vi "DAQInit.vi"(6 "Scan/Meas Parameters":T5={"Pixel Dwell Time (s)"=0.0001, "Pixel Size"=200.0, "X Min (V)"=-7.5, "X Max (V)"=7.5, "Y Min (V)"=-7.5, "Y Max (V)"=7.5, "XY Factor (1/V)"=0.2}, 7 "Calibration Parameters":T4={"Target Lifetime (s)"=4e-09, "Integration Time (s)"=0.1, "Calibration Steps"=500.0}, 8 "error in":errorcluster, 9 "Functions":T6(ring)=enum."Measurement", 10 "Global Parameters":T1={"DC AI Min (V)"=0.0015, "DC AI Max (V)"=0.06, "Mixer AI Min (V)"=-0.3, "Mixer AI Max (V)"=0.3, "Bias AO Min (V)"=-1.0, "Bias AO Max (V)"=7.0, "Scan AO Min (V)"=-10.0, "Scan AO Max (V)"=10.0, "Fast Samp Freq (Hz)"=2500000.0, "Slow Samp Freq (Hz)"=250000.0}, 11 "DAQ Channels":T3) -> (0 "error out":errorcluster, 2 "Expected Time (s)":dbl=98.154, 3 "Tasks Out":T2)   [LabVIEW 2015]
uses:
  <vilib>/DAQmx/create/channels.llb/DAQmx Create Channel (AO-Voltage-Basic).vi
  <vilib>/DAQmx/configure/timing.llb/DAQmx Timing (Sample Clock).vi
  <vilib>/DAQmx/create/channels.llb/DAQmx Create Channel (AI-Voltage-Basic).vi
  <vilib>/DAQmx/configure/trigger.llb/DAQmx Start Trigger (Digital Edge).vi
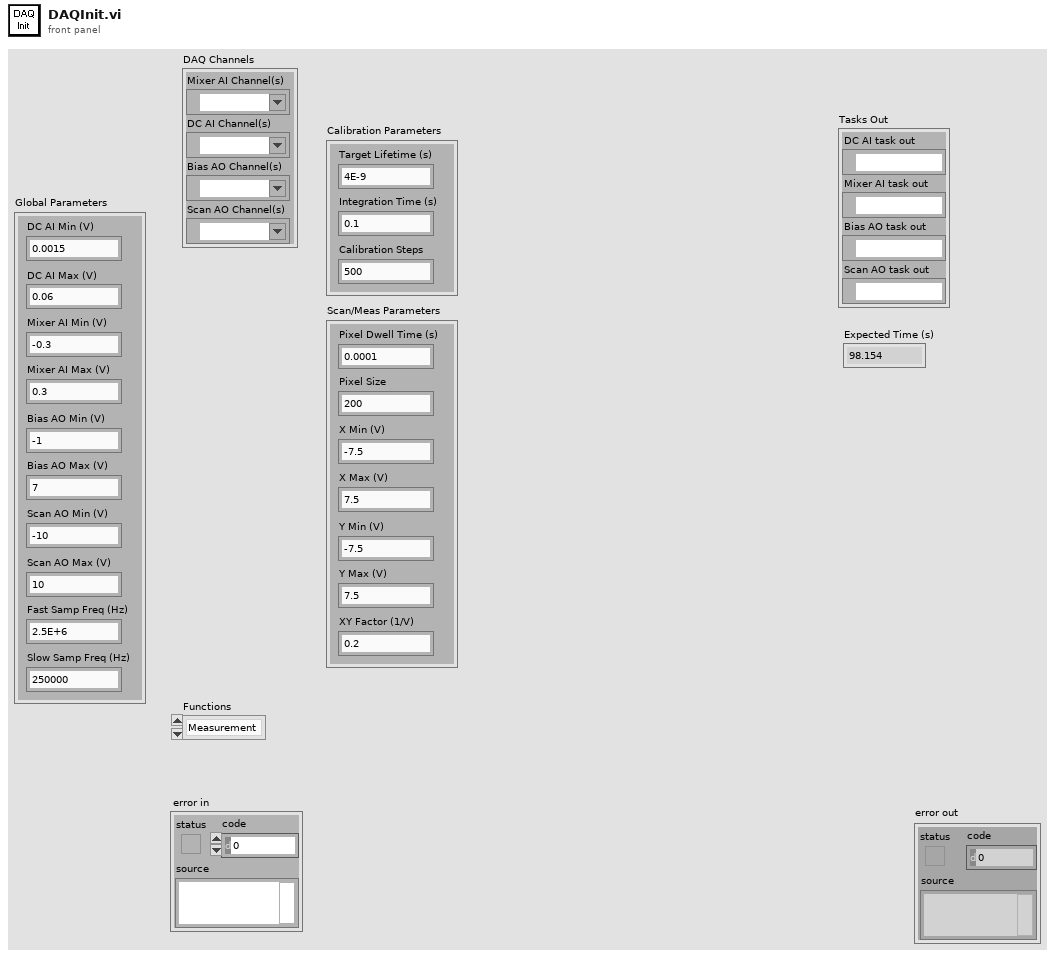
[diagram p1: front panel]
types:
  T1 = cluster{"DC AI Min (V)":dbl, "DC AI Max (V)":dbl, "Mixer AI Min (V)":dbl, "Mixer AI Max (V)":dbl, "Bias AO Min (V)":dbl, "Bias AO Max (V)":dbl, "Scan AO Min (V)":dbl, "Scan AO Max (V)":dbl, "Fast Samp Freq (Hz)":dbl, "Slow Samp Freq (Hz)":dbl}
  T2 = cluster{"DC AI task out":refnum<k21>, "Mixer AI task out":refnum<k21>, "Bias AO task out":refnum<k21>, "Scan AO task out":refnum<k21>}
  T3 = cluster{"Mixer AI Channel(s)":tag, "DC AI Channel(s)":tag, "Bias AO Channel(s) ":tag, "Scan AO Channel(s)":tag}
  T4 = cluster{"Target Lifetime (s)":dbl, "Integration Time (s)":dbl, "Calibration Steps":dbl}
  T5 = cluster{"Pixel Dwell Time (s)":dbl, "Pixel Size":dbl, "X Min (V)":dbl, "X Max (V)":dbl, "Y Min (V)":dbl, "Y Max (V)":dbl, "XY Factor (1/V)":dbl}
  T6 = enum32{"Calibration", "Fast Scan", "Measurement"}
  T7 = cluster{"task out":refnum<k21>, "task out":refnum<k21>, "task out":refnum<k21>, "task out":refnum<k21>}
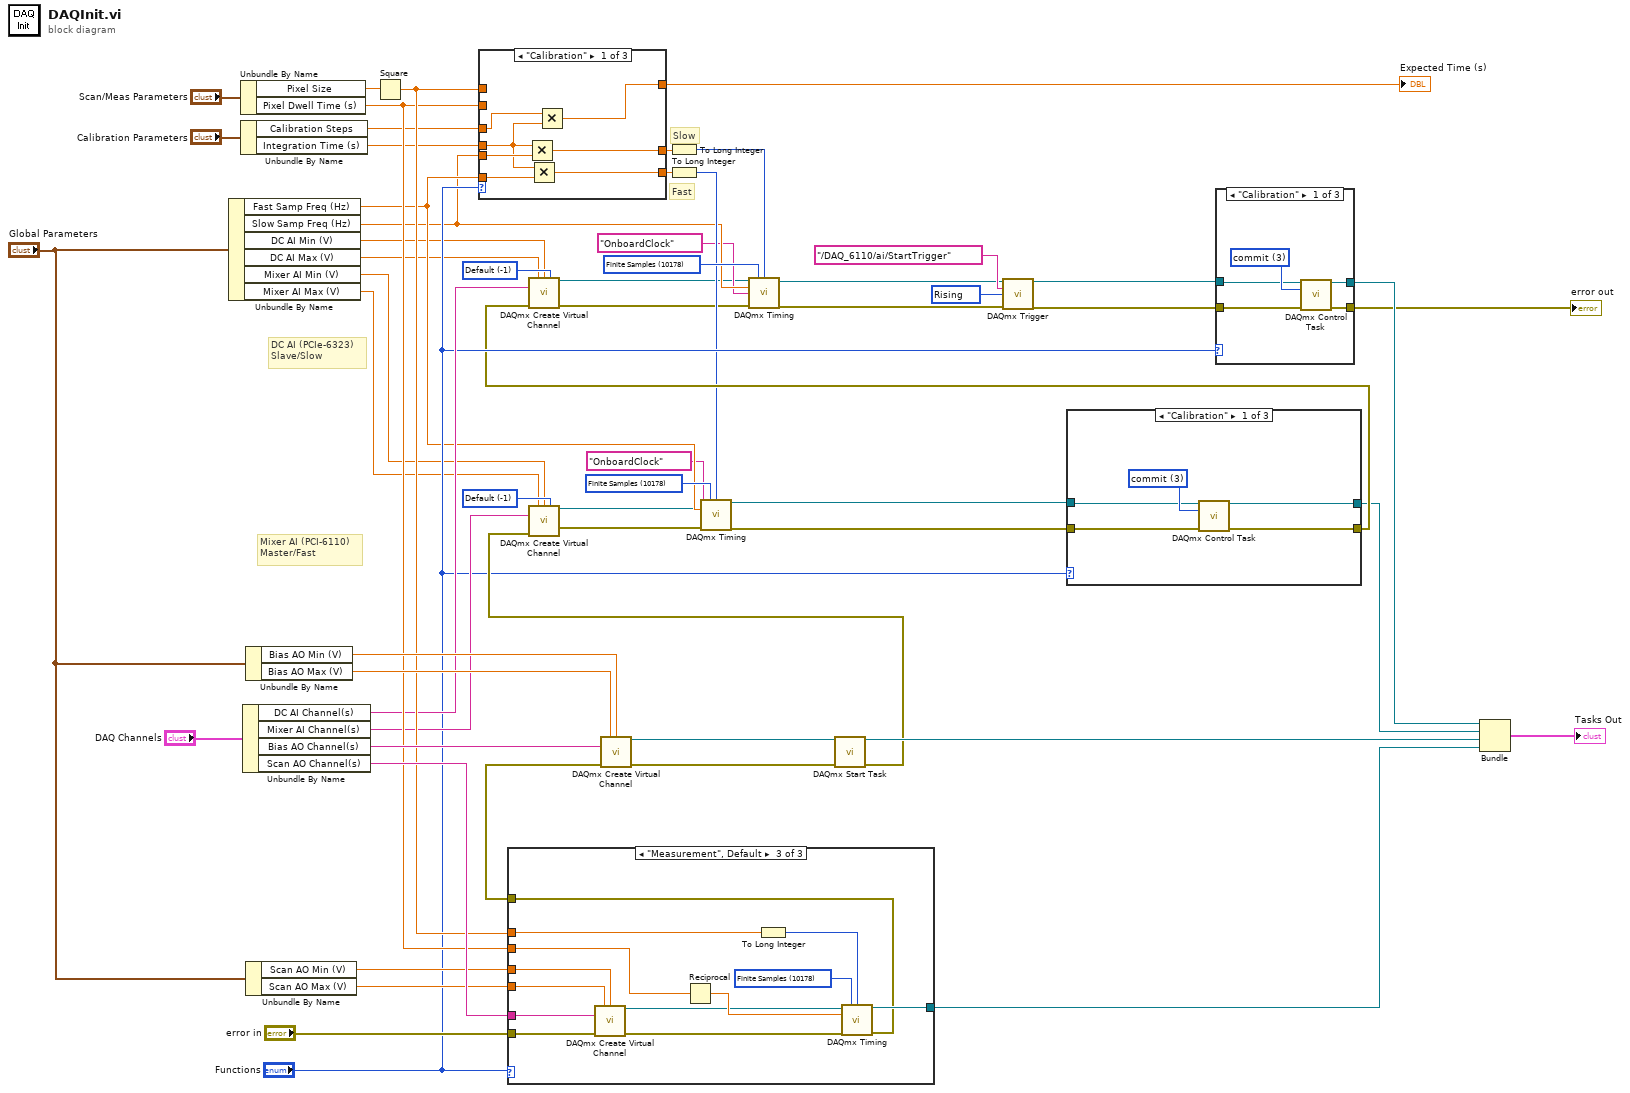
[diagram p0: block diagram]
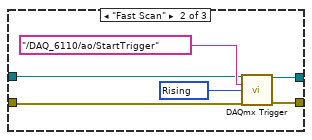
[diagram p2: hidden frame]
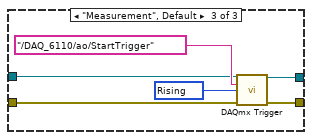
[diagram p3: hidden frame]
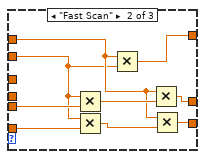
[diagram p4: hidden frame]
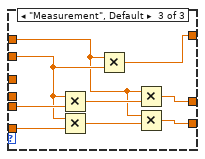
[diagram p5: hidden frame]
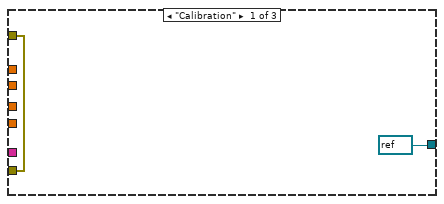
[diagram p8: hidden frame]
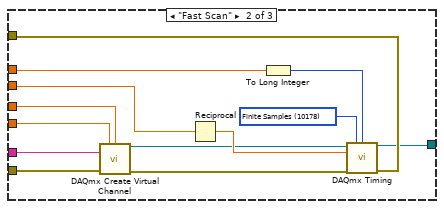
[diagram p9: hidden frame]
diagram:
  w13 = 10280 items=["Rising"=10280, "Falling"=10171] ("edge")
  w34 = 10178 items=["Finite Samples"=10178, "Continuous Samples"=10123, "Hardware Timed Single Point"=12522] ("sample mode")
  w35 = -1 items=["Default"=-1, "RSE"=10083, "NRSE"=10078, "Differential"=10106, "Pseudodifferential"=12529] ("input terminal configuration")
  w43 = 10178 items=["Finite Samples"=10178, "Continuous Samples"=10123, "Hardware Timed Single Point"=12522] ("sample mode")
  w44 = -1 items=["Default"=-1, "RSE"=10083, "NRSE"=10078, "Differential"=10106, "Pseudodifferential"=12529] ("input terminal configuration")
  # "Fast"
  # "Slow"
  # "DC AI (PCIe-6323)\nSlave/Slow"
  # "Mixer AI (PCI-6110)\nMaster/Fast"
  n1 = Unbundle By Name("Global Parameters") -> ("Fast Samp Freq (Hz)"=w24:dbl, "Slow Samp Freq (Hz)"=w20:dbl, "DC AI Min (V)"=w4:dbl, "DC AI Max (V)"=w2:dbl, "Mixer AI Min (V)"=w3:dbl, "Mixer AI Max (V)"=w1:dbl)
  n2 = Unbundle By Name("Scan/Meas Parameters") -> ("Pixel Size"=w53:dbl, "Pixel Dwell Time (s)"=w41:dbl)
  n3 = Unbundle By Name("Calibration Parameters") -> ("Calibration Steps"=w37:dbl, "Integration Time (s)"=w39:dbl)
  n4 = Unbundle By Name("DAQ Channels") -> ("DC AI Channel(s)"=w31:tag, "Mixer AI Channel(s)"=w32:tag, "Bias AO Channel(s)"=w48:tag, "Scan AO Channel(s)"=w56:tag)
  n5 = Unbundle By Name("Global Parameters") -> ("Bias AO Min (V)"=w46:dbl, "Bias AO Max (V)"=w47:dbl)
  n6 = Unbundle By Name("Global Parameters") -> ("Scan AO Min (V)"=w54:dbl, "Scan AO Max (V)"=w55:dbl)
  n7 = Square(x=w53) -> (x^2=w42:dbl)
  n8 = case shown="\"Calibration\"" "Functions" {
    tunnel: w20 -> [w66 w70 w83]
    tunnel: w42 -> [_ w71 w76]
    tunnel: w41 -> [_ w68 w79]
    tunnel: [w65 w74 w82] -> w40
    tunnel: w39 -> [w62 _ _]
    tunnel: [w63 w73 w81] -> w38
    tunnel: w37 -> [w64 _ _]
    tunnel: w24 -> [w61 w69 w80]
    tunnel: [w60 w72 w78] -> w26
    frame "Calibration" {
      n9 = Multiply(x=w62, y=w66) -> (x*y=w65:dbl)
      n10 = Multiply(x=w62, y=w61) -> (x*y=w60:dbl)
      n11 = Multiply(x=w64, y=w62) -> (x*y=w63:dbl)
    }
    frame "Fast Scan" {
      n12 = Multiply(x=w68, y=w70) -> (x*y=w75:dbl)
      n13 = Multiply(x=w68, y=w69) -> (x*y=w67:dbl)
      n14 = Multiply(x=w71, y=w68) -> (x*y=w73:dbl)
      n15 = Multiply(x=w71, y=w75) -> (x*y=w74:dbl)
      n16 = Multiply(x=w71, y=w67) -> (x*y=w72:dbl)
    }
    frame "Measurement", Default {
      n17 = Multiply(x=w79, y=w83) -> (x*y=w84:dbl)
      n18 = Multiply(x=w79, y=w80) -> (x*y=w77:dbl)
      n19 = Multiply(x=w76, y=w79) -> (x*y=w81:dbl)
      n20 = Multiply(x=w76, y=w84) -> (x*y=w82:dbl)
      n21 = Multiply(x=w76, y=w77) -> (x*y=w78:dbl)
    }
  }
  "Expected Time (s)" <- w38
  n22 = case shown="\"Measurement\", Default" "Functions" {
    tunnel: "error in" -> [w86 w88 w112]
    tunnel: w56 -> [_ w89 w111]
    tunnel: w55 -> [_ w90 w110]
    tunnel: w54 -> [_ w91 w109]
    tunnel: w41 -> [_ w92 w103]
    tunnel: w42 -> [_ w93 w102]
    tunnel: [refnum<k21> refnum ("task out") w87 w101] -> w52
    tunnel: [w86 w94 w100] -> w49
    frame "Calibration" {
    }
    frame "Fast Scan" {
      w99 = 10178 items=["Finite Samples"=10178, "Continuous Samples"=10123, "Hardware Timed Single Point"=12522] ("sample mode")
      n23 = call-poly <vilib>:"DAQmx Create Virtual Channel.vi"("maximum value"=w90, "minimum value"=w91, "physical channels"=w89, "error in"=w88) -> ("task out"=w96:refnum<k21>, "error out"=w95:errorcluster)  [unwired: 10 in]
      n24 = Reciprocal(x=w92) -> (1/x=w98:dbl)
      n25 = To Long Integer(number=w93) -> (32bit integer=w97:i32)
      n26 = call-poly <vilib>:"DAQmx Timing.vi"("task/channels in"=w96, "sample mode"=w99, "samples per channel"=w97, "rate"=w98, "error in"=w95) -> ("task out"=w87:refnum<k21>, "error out"=w94:errorcluster)  [unwired: 9 in]
    }
    frame "Measurement", Default {
      w108 = 10178 items=["Finite Samples"=10178, "Continuous Samples"=10123, "Hardware Timed Single Point"=12522] ("sample mode")
      n27 = call-poly <vilib>:"DAQmx Create Virtual Channel.vi"("maximum value"=w110, "minimum value"=w109, "physical channels"=w111, "error in"=w112) -> ("task out"=w105:refnum<k21>, "error out"=w104:errorcluster)  [unwired: 10 in]
      n28 = Reciprocal(x=w103) -> (1/x=w107:dbl)
      n29 = To Long Integer(number=w102) -> (32bit integer=w106:i32)
      n30 = call-poly <vilib>:"DAQmx Timing.vi"("task/channels in"=w105, "sample mode"=w108, "samples per channel"=w106, "rate"=w107, "error in"=w104) -> ("task out"=w101:refnum<k21>, "error out"=w100:errorcluster)  [unwired: 9 in]
    }
  }
  n31 = call-poly <vilib>:"DAQmx Create Virtual Channel.vi"("maximum value"=w47, "minimum value"=w46, "physical channels"=w48, "error in"=w49) -> ("task out"=w51:refnum<k21>, "error out"=w50:errorcluster)  [unwired: 10 in]
  n32 = To Long Integer(number=w40) -> (32bit integer=w29:i32)
  n33 = To Long Integer(number=w26) -> (32bit integer=w25:i32)
  n34 = call <vilib>:"DAQmx Start Task.vi"("task/channels in"=w51, "error in"=w50) -> ("task out"=w45:refnum<k21>, "error out"=w33:errorcluster)  [unwired: 12 in]
  n35 = call-poly <vilib>:"DAQmx Create Virtual Channel.vi"("maximum value"=w1, "minimum value"=w3, "input terminal configuration"=w35, "physical channels"=w32, "error in"=w33) -> ("task out"=w23:refnum<k21>, "error out"=w22:errorcluster)  [unwired: 9 in]
  n36 = call-poly <vilib>:"DAQmx Timing.vi"("task/channels in"=w23, "sample mode"=w34, "samples per channel"=w25, "rate"=w24, "source"=tag "OnboardClock", "error in"=w22) -> ("task out"=w17:refnum<k21>, "error out"=w16:errorcluster)  [unwired: 8 in]
  n37 = case shown="\"Calibration\"" "Functions" {
    tunnel: w16 -> [w115 w120 w127]
    tunnel: w17 -> [w116 w121 w126]
    tunnel: [w114 w119 w125] -> w28
    tunnel: [w113 w118 w124] -> w21
    frame "Calibration" {
      w117 = 3 items=["verify"=2, "reserve"=4, "commit"=3, "unreserve"=5, "abort"=6] ("action")
      n38 = call <vilib>:"DAQmx Control Task.vi"("task/channels in"=w116, "action"=w117, "error in"=w115) -> ("task out"=w113:refnum<k21>, "error out"=w114:errorcluster)  [unwired: 11 in]
    }
    frame "Fast Scan" {
      w123 = 10280 items=["Rising"=10280, "Falling"=10171] ("edge")
      n39 = call-poly <vilib>:"DAQmx Trigger.vi"("task/channels in"=w121, "source"=tag "/DAQ_6110/ao/StartTrigger", "edge"=w123, "error in"=w120) -> ("task out"=w118:refnum<k21>, "error out"=w119:errorcluster)  [unwired: 10 in]
    }
    frame "Measurement", Default {
      w128 = 10280 items=["Rising"=10280, "Falling"=10171] ("edge")
      n40 = call-poly <vilib>:"DAQmx Trigger.vi"("task/channels in"=w126, "source"=tag "/DAQ_6110/ao/StartTrigger", "edge"=w128, "error in"=w127) -> ("task out"=w124:refnum<k21>, "error out"=w125:errorcluster)  [unwired: 10 in]
    }
  }
  n41 = call-poly <vilib>:"DAQmx Create Virtual Channel.vi"("maximum value"=w2, "minimum value"=w4, "input terminal configuration"=w44, "physical channels"=w31, "error in"=w28) -> ("task out"=w15:refnum<k21>, "error out"=w14:errorcluster)  [unwired: 9 in]
  n42 = call-poly <vilib>:"DAQmx Timing.vi"("task/channels in"=w15, "sample mode"=w43, "samples per channel"=w29, "rate"=w20, "source"=tag "OnboardClock", "error in"=w14) -> ("task out"=w9:refnum<k21>, "error out"=w6:errorcluster)  [unwired: 8 in]
  n43 = call-poly <vilib>:"DAQmx Trigger.vi"("task/channels in"=w9, "source"=tag "/DAQ_6110/ai/StartTrigger", "edge"=w13, "error in"=w6) -> ("task out"=w8:refnum<k21>, "error out"=w7:errorcluster)  [unwired: 10 in]
  n44 = case shown="\"Calibration\"" "Functions" {
    tunnel: w7 -> [w132 w135 w137]
    tunnel: w8 -> [w133 w136 w138]
    tunnel: [w131 w135 w137] -> w10
    tunnel: [w130 w136 w138] -> w11
    frame "Calibration" {
      w134 = 3 items=["verify"=2, "reserve"=4, "commit"=3, "unreserve"=5, "abort"=6] ("action")
      n45 = call <vilib>:"DAQmx Control Task.vi"("task/channels in"=w133, "action"=w134, "error in"=w132) -> ("task out"=w130:refnum<k21>, "error out"=w131:errorcluster)  [unwired: 11 in]
    }
    frame "Fast Scan" {
    }
    frame "Measurement", Default {
    }
  }
  "error out" <- w10
  n46 = Bundle("task out"=w11, "task out"=w21, "task out"=w45, "task out"=w52) -> (→"Tasks Out":T7)  [unwired: 1 in]
